vi "denomination(SubVI).vi"(1 "Enter Amount":i32 min=100 max=100000 step=100) -> (0 "String":string)   [LabVIEW 2020]
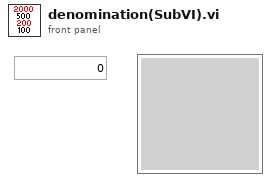
[diagram p1: front panel]
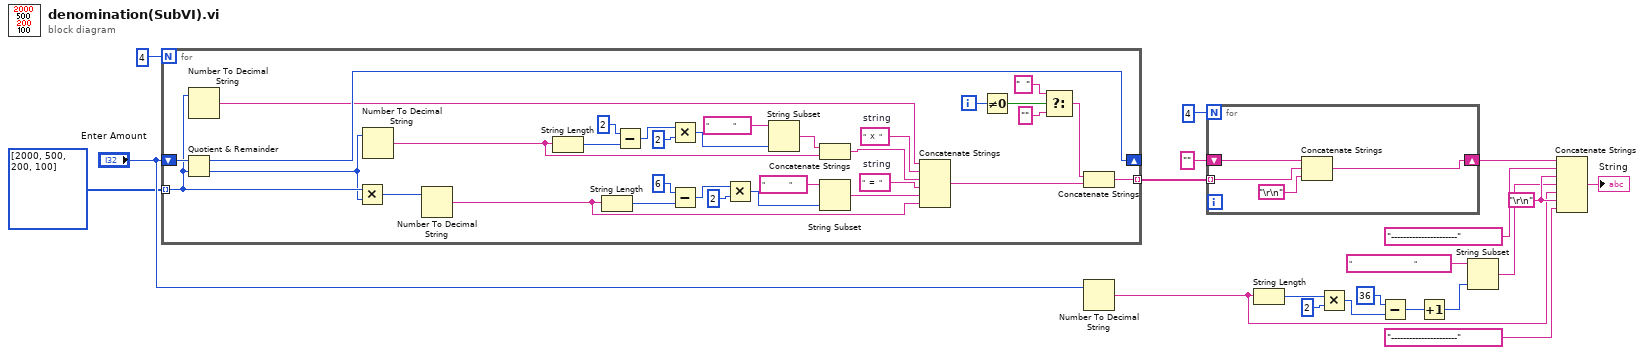
[diagram p0: block diagram]
diagram:
  w19 = "\r\n"
  n1 = for {
    N: 4 -> [_]
    tunnel: i32[] [2000, 500, 200, 100] -> [w47] mode=indexing
    shift-right: [w51] -> _
    shift-left: "Enter Amount" -> [w52]
    tunnel: [w40] -> w13 mode=indexing
    i -> [w39]
    w48 = "  =  "  # string
    w49 = "  X  "  # string
    n2 = Quotient & Remainder(x=w52, y=w47) -> (x-y*floor(x/y)=w51:i32, floor(x/y)=w36:i32)
    n3 = Number To Decimal String(number=w47) -> (decimal integer string=w50:string)  [unwired: 1 in]
    n4 = Multiply(x=w47, y=w36) -> (x*y=w46:i32)
    n5 = Number To Decimal String(number=w36) -> (decimal integer string=w22:string)  [unwired: 1 in]
    n6 = Number To Decimal String(number=w46) -> (decimal integer string=w34:string)  [unwired: 1 in]
    n7 = String Length(string=w22) -> (length=w29:i32)
    n8 = String Length(string=w34) -> (length=w38:i32)
    n9 = Subtract(x=2, y=w29) -> (x-y=w27:i32)
    n10 = Multiply(x=w27, y=2) -> (x*y=w24:i32)
    n11 = Subtract(x=6, y=w38) -> (x-y=w32:i32)
    n12 = Multiply(x=w32, y=2) -> (x*y=w31:i32)
    n13 = String Subset(string="            ", length (rest)=w24) -> (substring=w23:string)  [unwired: 1 in]
    n14 = Concatenate Strings(w23, w22) -> (w21:string)
    n15 = String Subset(string="            ", length (rest)=w31) -> (substring=w33:string)  [unwired: 1 in]
    n16 = Concatenate Strings "Concatenate Strings"(w50, w49, w21, w48, w33, w34) -> (w41:string)
    n17 = Not Equal To 0?(x=w39) -> (x != 0?=w45:bool)
    n18 = Select(t="  ", s=w45, f="") -> (s? t:f=w42:string)
    n19 = Concatenate Strings(w42, w41) -> (w40:string)
  }
  n20 = Number To Decimal String(number="Enter Amount") -> (decimal integer string=w11:string)  [unwired: 1 in]
  n21 = for {
    N: 4 -> [_]
    tunnel: w13 -> [w54] mode=indexing
    shift-right: [w56] -> w16
    shift-left: "" -> [w53]
    n22 = Concatenate Strings "Concatenate Strings"(w53, w54, "\r\n") -> (w56:string)
  }
  n23 = String Length(string=w11) -> (length=w2:i32)
  n24 = Multiply(x=w2, y=2) -> (x*y=w3:i32)
  n25 = Subtract(x=36, y=w3) -> (x-y=w5:i32)
  n26 = Increment(x=w5) -> (x+1=w1:i32)
  n27 = String Subset(string="                               ", length (rest)=w1) -> (substring=w8:string)  [unwired: 1 in]
  n28 = Concatenate Strings(w16, "----------------------" ("string"), w19, w8, w11, w19, "----------------------" ("string")) -> (→"String":string)
